vi "Get Log File Pretrigger Logging.vi"(8 "error in":errorcluster, 11 "log file in":T1 format="%.0x") -> (0 "error out":errorcluster, 1 "pretrigger samples":i32, 2 "pretrigger logging":bool, 3 "log file out":T1 format="%.0x")   [LabVIEW 2027, in "Embedded Data Logger Scripting.lvlib"]
uses:
  Embedded Data Logger Scripting.lvlib
  <vilib>/NI VeriStand/Custom Device API/Custom Device Item Ref.ctl
  <vilib>/NI VeriStand/Custom Device API/Get Item Property (Boolean).vi
  <vilib>/NI VeriStand/Custom Device API/Get Item Property (I32).vi
  <vilib>/NI VeriStand/Custom Device API/Custom Device API.lvlib
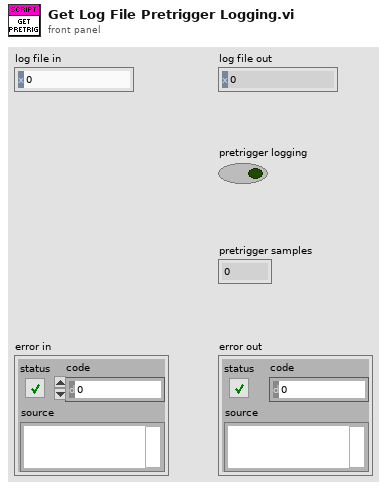
[diagram p1: front panel]
types:
  T1 = typedef "Custom Device API.lvlib/Custom Device Item Ref.ctl" = u64
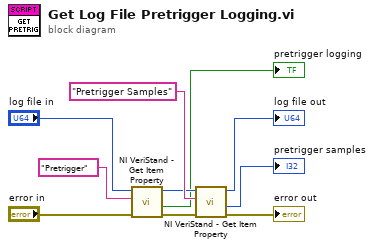
[diagram p0: block diagram]
diagram:
  n1 = call-poly <vilib>:"NI VeriStand - Get Item Property.vi"("error in (no error)"="error in", "Property Name"="Pretrigger", "Item Ref in"="log file in") -> ("error out"=w7:errorcluster, "Value"=→"pretrigger logging":bool, "Item Ref out"=w5:T1)  [unwired: 5 in, 1 out]
  n2 = call-poly <vilib>:"NI VeriStand - Get Item Property.vi"("error in (no error)"=w7, "Property Name"="Pretrigger Samples", "Item Ref in"=w5) -> ("error out"=→"error out":errorcluster, "Value"=→"pretrigger samples":i32, "Item Ref out"=→"log file out":T1)  [unwired: 5 in, 1 out]
